vi "Scale_Offset_Pan.vi"(8 "error in (no error)":errorcluster caption="entrée d'erreur (pas d'erreur)") -> (0 "error out":errorcluster caption="sortie d'erreur")   [LabVIEW 2019]
panel:
  out "EdPan Cluster Out":T1
  in  "EdPan Cluster":T1={"X Offset"=0.0, "Y Offset"=0.0, "X Scale"=1.0, "Y Scale"=1.0} {"Y Scale" min=0.1 step=0.1 format="%#.3f"; "X Scale" min=0.1 step=0.1 format="%#.3f"; "Y Offset" format="%.3f"; "X Offset" format="%.3f"}
  out "EdPanelName":string="Scale & Offset"
  out "X Data Out":dbl[][](array[numeric])
  in  "XData":dbl[][](array[numeric])
  out "Y Data Out":dbl[][](array[numeric])
  in  "YData":dbl[][](array[numeric])
  in  "Apply_to":enum16{"X Data", "Y Data"}(ring) caption="Apply to:"
  in  "Quick Scale":dbl(slide) scale=0.0..6.0
  in  "Quick Offset":dbl(slide) scale=0.0..4.0
  in  "EditorProgQ":refnum<queue>
  in  "EditorProgQEvent":refnum<user-event>
  in  "Stop":bool
  in  "Offset":dbl format="%.3f"
  in  "Scale":dbl=60.0 format="%#.3f"
  out "Init Program":bool
  # "this MUST be present and labeled \"Stop\""
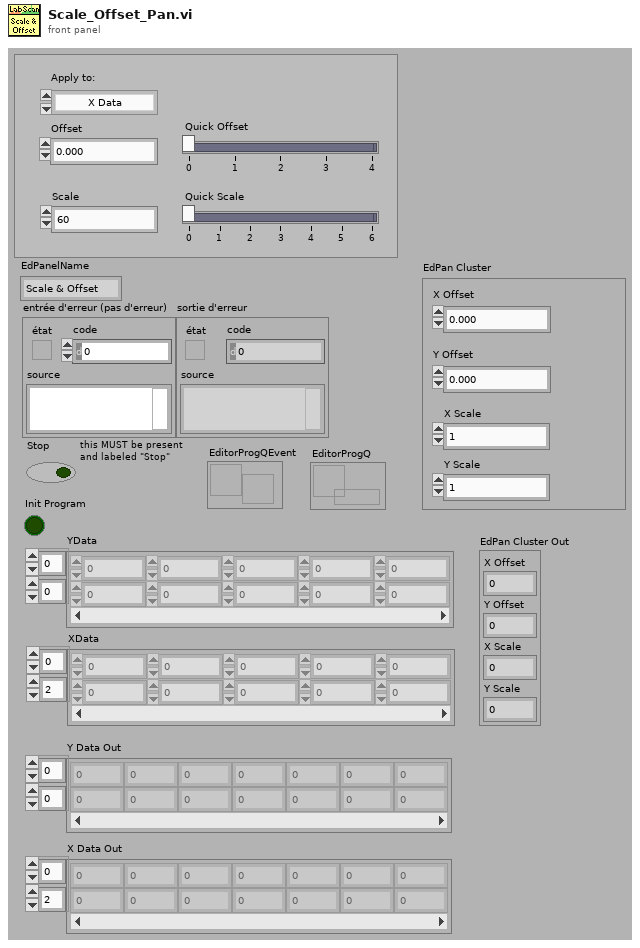
[diagram p1: front panel]
types:
  T1 = cluster{"X Offset":dbl, "Y Offset":dbl, "X Scale":dbl, "Y Scale":dbl}
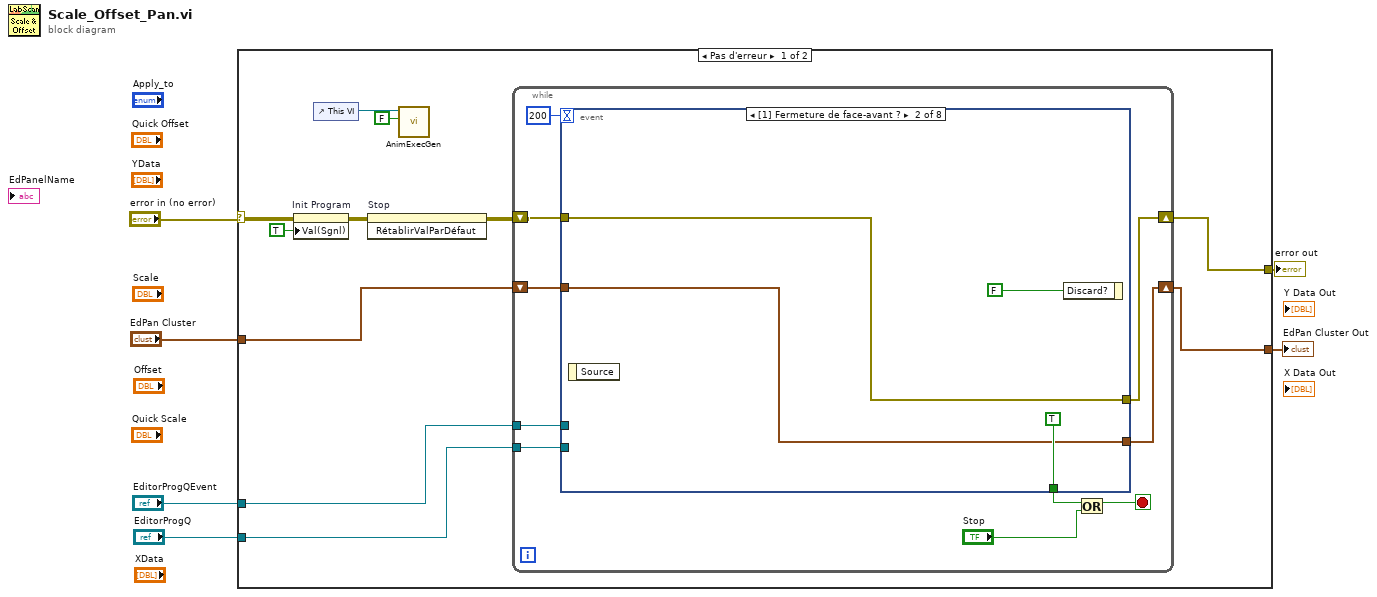
[diagram p0: block diagram]
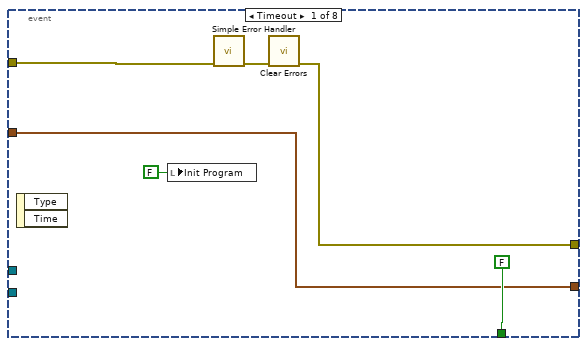
[diagram p2: hidden frame]
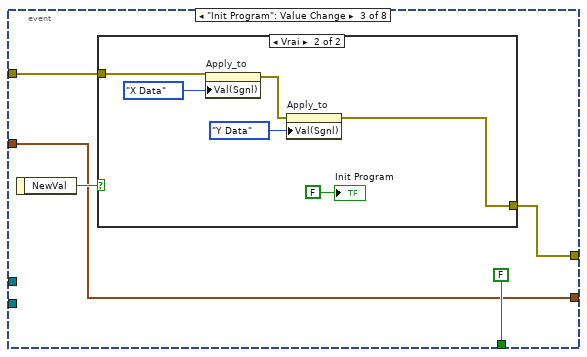
[diagram p3: hidden frame]
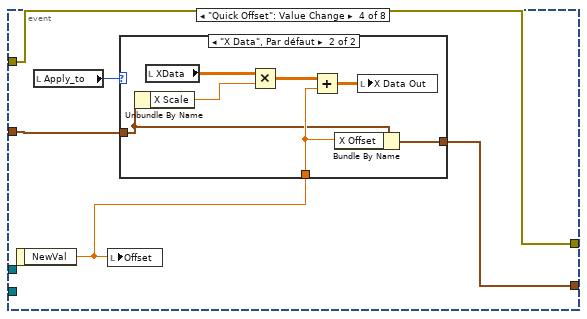
[diagram p5: hidden frame]
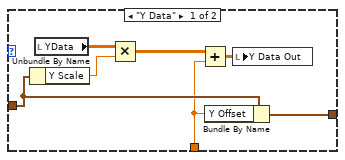
[diagram p6: hidden frame]
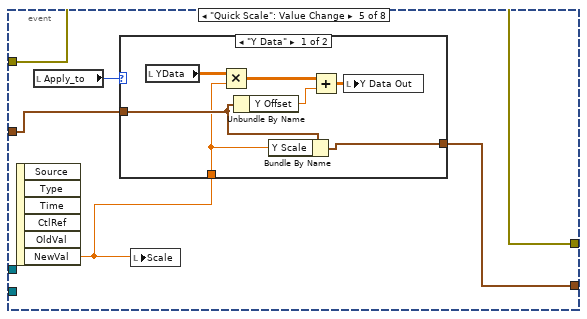
[diagram p7: hidden frame]
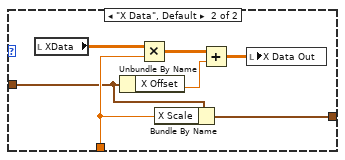
[diagram p8: hidden frame]
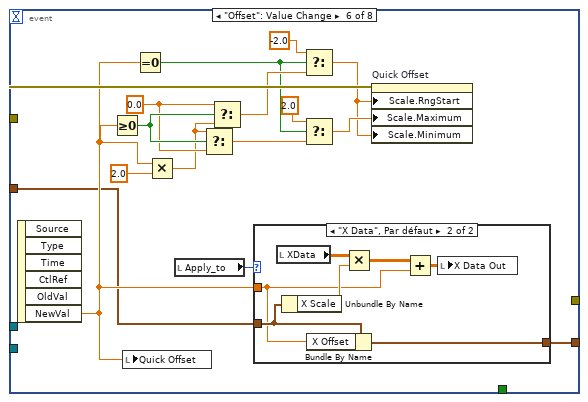
[diagram p9: hidden frame]
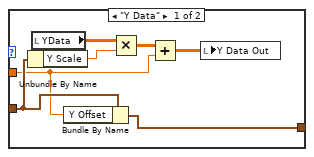
[diagram p10: hidden frame]
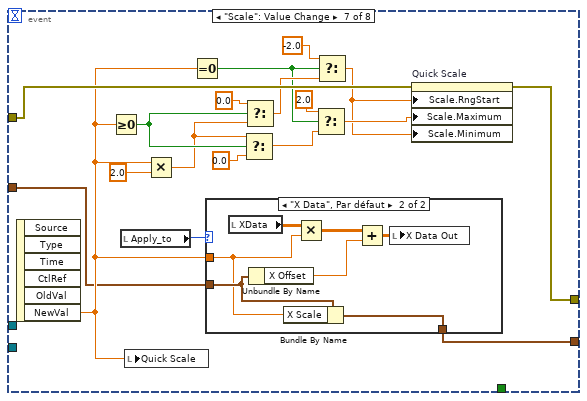
[diagram p11: hidden frame]
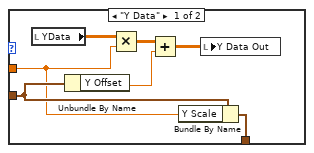
[diagram p12: hidden frame]
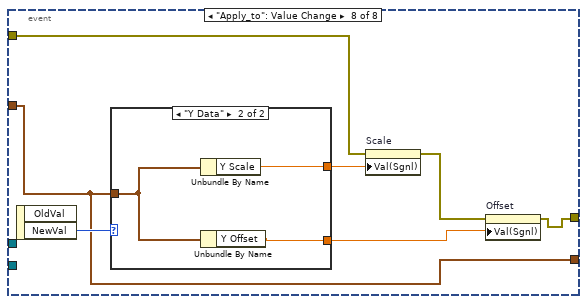
[diagram p13: hidden frame]
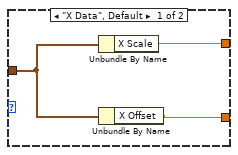
[diagram p14: hidden frame]
diagram:
  n1 = case shown="Pas d'erreur" "error in (no error)" {
    selector: "error in (no error)" -> [w15 w164]
    tunnel: [w17 w164] -> w5
    tunnel: "EditorProgQEvent" -> [w10 _]
    tunnel: "EditorProgQ" -> [w9 _]
    tunnel: "EdPan Cluster" -> [w8 w163]
    tunnel: [w7 w163] -> w1
    frame No Error {
      n2 = property on="Init Program" class="Bool (strict)"(error in=w15, "Val(Sgnl)"=TRUE ("Valeur (Signalisation)")) -> (error out=w14:errorcluster)  [unwired: 1 in, 1 out]
      n3 = control-ref of="This VI"() -> (w11:refnum<vi>)
      n4 = invoke on="Stop" class="Bool (strict)" method="RétablirValParDéfaut"(error in=w14) -> (error out=w13:errorcluster)  [unwired: 2 in, 2 out]
      n5 = call <userlib>:"AnimExecGen.vi"("Animer l'exécution ?"=FALSE, "ViRef"=w11) -> ()  [unwired: 9 in, 1 out]
      n6 = while {
        shift-right: [w25] -> w17
        shift-left: w13 -> [w26]
        tunnel: w10 -> [w21]
        tunnel: w9 -> [w20]
        shift-right: [w18] -> w7
        shift-left: w8 -> [w19]
        stop <- w23 stop-if-true
        n7 = event shown="[1] Fermeture de face-avant ?" {
          selector: _ -> [_ _ _ _ _ _ _ _]
          dyn-events: _ -> [_ _ _ _ _ _ _ _]
          timeout: 200 -> [_ _ _ _ _ _ _ _]
          tunnel: w26 -> [w32 w35 w41 w50 w69 w103 w135 w156]
          tunnel: [w30 w35 w40 w50 w69 _ w128 w151] -> w25
          tunnel: [FALSE TRUE FALSE _ _ _ _ _] -> w24
          tunnel: w21 -> [_ _ _ _ _ _ _ _]
          tunnel: w20 -> [_ _ _ _ _ _ _ _]
          tunnel: w19 -> [w28 w34 w38 w52 w71 w89 w119 w150]
          tunnel: [w28 w34 w38 w51 w70 w88 w118 w150] -> w18
          event Timeout {
            n8 = event-data() -> ()  [unwired: 1 in, 2 out]
            n9 = local write "Init Program"(FALSE ("Init Program")) -> ()
            n10 = call <vilib>:"Simple Error Handler.vi"("error in (no error)"=w32) -> ("error out"=w31:errorcluster)  [unwired: 4 in, 4 out]
            n11 = call <vilib>:"Clear Errors.vi"("error in (no error)"=w31) -> ("error out"=w30:errorcluster)  [unwired: 5 in, 1 out]
          }
          event Panel Close? {
            n12 = event-data() -> ()  [unwired: 1 in, 1 out]
            n13 = event-data("Discard?"=FALSE ("Rejeter ?")) -> ()  [unwired: 1 in, 1 out]
          }
          event "Init Program": Value Change {
            n14 = event-data() -> ("NewVal"=w42:bool)  [unwired: 1 in]
            n15 = case shown="Vrai" w42 {
              tunnel: w41 -> [w43 w46]
              tunnel: [w43 w48] -> w40
              frame False {
              }
              frame True {
                n16 = property on="Apply_to" class="Énum (strict)"(error in=w46, "Val(Sgnl)"=enum16{"X Data", "Y Data"}."X Data" ("Valeur (Signalisation)")) -> (error out=w45:errorcluster)  [unwired: 1 in, 1 out]
                n17 = property on="Apply_to" class="Énum (strict)"(error in=w45, "Val(Sgnl)"=enum16{"X Data", "Y Data"}."Y Data" ("Valeur (Signalisation)")) -> (error out=w48:errorcluster)  [unwired: 1 in, 1 out]
                "Init Program" <- FALSE
              }
            }
          }
          event "Quick Offset": Value Change {
            n18 = event-data() -> ("NewVal"=w54:dbl)  [unwired: 1 in]
            n19 = local read "Apply_to"() -> (w53:enum16{"X Data", "Y Data"})
            n20 = local write "Offset"(w54) -> ()
            n21 = case shown="\"X Data\", Par défaut" w53 {
              tunnel: w54 -> [w56 w64]
              tunnel: w52 -> [w57 w63]
              tunnel: [w55 w62] -> w51
              frame "Y Data" {
                n22 = Unbundle By Name(w57) -> ("Y Scale"=w58:dbl)
                n23 = local read "YData"() -> (w59:dbl[][])
                n24 = Multiply(x=w59, y=w58) -> (x*y=w60:dbl[][])
                n25 = Add(x=w60, y=w56) -> (x+y=w61:dbl[][])
                n26 = Bundle By Name(cluster=w57, "Y Offset"=w56) -> (w55:T1)
                n27 = local write "Y Data Out"(w61) -> ()
              }
              frame "X Data", Default {
                n28 = Unbundle By Name(w63) -> ("X Scale"=w65:dbl)
                n29 = local read "XData"() -> (w68:dbl[][])
                n30 = Multiply(x=w68, y=w65) -> (x*y=w66:dbl[][])
                n31 = Add(x=w66, y=w64) -> (x+y=w67:dbl[][])
                n32 = Bundle By Name(cluster=w63, "X Offset"=w64) -> (w62:T1)
                n33 = local write "X Data Out"(w67) -> ()
              }
            }
          }
          event "Quick Scale": Value Change {
            n34 = event-data() -> ("NewVal"=w73:dbl)  [unwired: 1 in, 5 out]
            n35 = local read "Apply_to"() -> (w72:enum16{"X Data", "Y Data"})
            n36 = case shown="\"Y Data\"" w72 {
              tunnel: w73 -> [w76 w83]
              tunnel: w71 -> [w77 w82]
              tunnel: [w74 w81] -> w70
              frame "Y Data" {
                n37 = local read "YData"() -> (w78:dbl[][])
                n38 = Multiply(x=w78, y=w76) -> (x*y=w79:dbl[][])
                n39 = Unbundle By Name(w77) -> ("Y Offset"=w75:dbl)
                n40 = Bundle By Name(cluster=w77, "Y Scale"=w76) -> (w74:T1)
                n41 = Add(x=w79, y=w75) -> (x+y=w80:dbl[][])
                n42 = local write "Y Data Out"(w80) -> ()
              }
              frame "X Data", Default {
                n43 = local read "XData"() -> (w87:dbl[][])
                n44 = Unbundle By Name(w82) -> ("X Offset"=w84:dbl)
                n45 = Multiply(x=w87, y=w83) -> (x*y=w85:dbl[][])
                n46 = Bundle By Name(cluster=w82, "X Scale"=w83) -> (w81:T1)
                n47 = Add(x=w85, y=w84) -> (x+y=w86:dbl[][])
                n48 = local write "X Data Out"(w86) -> ()
              }
            }
            n49 = local write "Scale"(w73) -> ()
          }
          event "Offset": Value Change {
            w101 = 0.0 ("cas vrai")
            n50 = event-data() -> ("NewVal"=w98:dbl)  [unwired: 1 in, 5 out]
            n51 = Greater Or Equal To 0?(x=w98) -> (x >= 0?=w102:bool)
            n52 = local write "Quick Offset"(w98) -> ()
            n53 = Equal To 0?(x=w98) -> (x = 0?=w95:bool)
            n54 = Multiply(x=w98, y=2.0) -> (x*y=w91:dbl)
            n55 = local read "Apply_to"() -> (w100:enum16{"X Data", "Y Data"})
            n56 = Select(t=w91, s=w102, f=w101) -> (s? t:f=w94:dbl)
            n57 = Select(t=w101, s=w102, f=w91) -> (s? t:f=w97:dbl)
            n58 = case shown="\"X Data\", Par défaut" w100 {
              tunnel: w98 -> [w104 w111]
              tunnel: w89 -> [w106 w113]
              tunnel: [w105 w112] -> w88
              frame "Y Data" {
                n59 = Unbundle By Name(w106) -> ("Y Scale"=w107:dbl)
                n60 = local read "YData"() -> (w108:dbl[][])
                n61 = Bundle By Name(cluster=w106, "Y Offset"=w104) -> (w105:T1)
                n62 = Multiply(x=w108, y=w107) -> (x*y=w109:dbl[][])
                n63 = Add(x=w109, y=w104) -> (x+y=w110:dbl[][])
                n64 = local write "Y Data Out"(w110) -> ()
              }
              frame "X Data", Default {
                n65 = local read "XData"() -> (w116:dbl[][])
                n66 = Unbundle By Name(w113) -> ("X Scale"=w114:dbl)
                n67 = Bundle By Name(cluster=w113, "X Offset"=w111) -> (w112:T1)
                n68 = Multiply(x=w116, y=w114) -> (x*y=w115:dbl[][])
                n69 = Add(x=w115, y=w111) -> (x+y=w117:dbl[][])
                n70 = local write "X Data Out"(w117) -> ()
              }
            }
            n71 = Select(t=-2.0 ("cas vrai"), s=w95, f=w97) -> (s? t:f=w90:dbl)
            n72 = Select(t=2.0 ("cas vrai"), s=w95, f=w94) -> (s? t:f=w93:dbl)
            n73 = property on="Quick Offset" class="Gliss (strict)"(error in=w103, "Scale.RngStart"=w90, "Scale.Maximum"=w93, "Scale.Minimum"=w90) -> ()  [unwired: 1 in, 2 out]
          }
          event "Scale": Value Change {
            n74 = event-data() -> ("NewVal"=w130:dbl)  [unwired: 1 in, 5 out]
            n75 = Greater Or Equal To 0?(x=w130) -> (x >= 0?=w134:bool)
            n76 = local read "Apply_to"() -> (w131:enum16{"X Data", "Y Data"})
            n77 = local write "Quick Scale"(w130) -> ()
            n78 = Multiply(x=w130, y=2.0) -> (x*y=w122:dbl)
            n79 = Equal To 0?(x=w130) -> (x = 0?=w127:bool)
            n80 = case shown="\"X Data\", Par défaut" w131 {
              tunnel: w130 -> [w137 w144]
              tunnel: w119 -> [w138 w146]
              tunnel: [w136 w143] -> w118
              frame "Y Data" {
                n81 = local read "YData"() -> (w140:dbl[][])
                n82 = Unbundle By Name(w138) -> ("Y Offset"=w139:dbl)
                n83 = Multiply(x=w140, y=w137) -> (x*y=w141:dbl[][])
                n84 = Add(x=w141, y=w139) -> (x+y=w142:dbl[][])
                n85 = Bundle By Name(cluster=w138, "Y Scale"=w137) -> (w136:T1)
                n86 = local write "Y Data Out"(w142) -> ()
              }
              frame "X Data", Default {
                n87 = local read "XData"() -> (w148:dbl[][])
                n88 = Unbundle By Name(w146) -> ("X Offset"=w145:dbl)
                n89 = Bundle By Name(cluster=w146, "X Scale"=w144) -> (w143:T1)
                n90 = Multiply(x=w148, y=w144) -> (x*y=w147:dbl[][])
                n91 = Add(x=w147, y=w145) -> (x+y=w149:dbl[][])
                n92 = local write "X Data Out"(w149) -> ()
              }
            }
            n93 = Select(t=w122, s=w134, f=0.0 ("cas vrai")) -> (s? t:f=w126:dbl)
            n94 = Select(t=0.0 ("cas vrai"), s=w134, f=w122) -> (s? t:f=w129:dbl)
            n95 = Select(t=2.0 ("cas vrai"), s=w127, f=w126) -> (s? t:f=w125:dbl)
            n96 = Select(t=-2.0 ("cas vrai"), s=w127, f=w129) -> (s? t:f=w120:dbl)
            n97 = property on="Quick Scale" class="Gliss (strict)"(error in=w135, "Scale.RngStart"=w120, "Scale.Maximum"=w125, "Scale.Minimum"=w120) -> (error out=w128:errorcluster)  [unwired: 1 in, 1 out]
          }
          event "Apply_to": Value Change {
            n98 = event-data() -> ("NewVal"=w155:enum16{"X Data", "Y Data"})  [unwired: 1 in, 1 out]
            n99 = case shown="\"Y Data\"" w155 {
              tunnel: [w157 w160] -> w154
              tunnel: [w158 w161] -> w152
              tunnel: w150 -> [w159 w162]
              frame "X Data", Default {
                n100 = Unbundle By Name(w159) -> ("X Scale"=w157:dbl)
                n101 = Unbundle By Name(w159) -> ("X Offset"=w158:dbl)
              }
              frame "Y Data" {
                n102 = Unbundle By Name(w162) -> ("Y Scale"=w160:dbl)
                n103 = Unbundle By Name(w162) -> ("Y Offset"=w161:dbl)
              }
            }
            n104 = property on="Scale" class="NumNb (strict)"(error in=w156, "Val(Sgnl)"=w154) -> (error out=w153:errorcluster)  [unwired: 1 in, 1 out]
            n105 = property on="Offset" class="NumNb (strict)"(error in=w153, "Val(Sgnl)"=w152) -> (error out=w151:errorcluster)  [unwired: 1 in, 1 out]
          }
        }
        n106 = Or(x=w24, y="Stop") -> (x .or. y?=w23:bool)
      }
    }
    frame Error {
    }
  }
  "error out" <- w5
  "EdPan Cluster Out" <- w1
